vi "Get Volume Free Space.vi"(11 "path":path) -> (2 "Current Free Space (kb)":dbl)   [LabVIEW 2013]
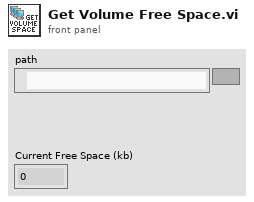
[diagram p1: front panel]
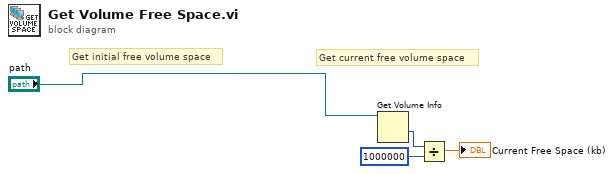
[diagram p0: block diagram]
diagram:
  # "Get current free volume space"
  # "Get initial free volume space"
  n1 = Get Volume Info(11:"path") -> (1:w3:i64)  [unwired: 1 in, 5 out]
  n2 = Divide(x=w3, y=i64 1000000) -> (x/y=→"Current Free Space (kb)":dbl)
